vi "Read Serial Interface.vi"(8 "error in":errorcluster, 11 "VISA Interface in":refnum<class "VISA Interface.lvclass">) -> (0 "error out":errorcluster, 2 "Serial Interface":T1={"Baud Rate"=9600, "Data Bits "=8, "Parity"=enum."None", "Stop Bits"=0} {"Stop Bits" items=["1.0", "1.5", "2.0"]; "Baud Rate" items=["1200"=1200, "2400"=2400, "4800"=4800, "9600"=9600, "19200"=19200, "38400"=38400, "57600"=57600, "115200"=115200]}, 3 "VISA Interface out":refnum<class "VISA Interface.lvclass">)   [LabVIEW 2020, in "Plugin Instrument Driver.lvlib" / "VISA Interface.lvclass"]
doc: "Reads Serial Interface"
uses:
  VISA Interface.lvclass
  builds/Libraries/Shared GUI Library.lvlibp/Shared GUI Library/Instrument Settings/Interface/Serial Interafce.ctl
  VISA Interface.lvclass/VISA Interface.ctl
  builds/Libraries/Shared GUI Library.lvlibp
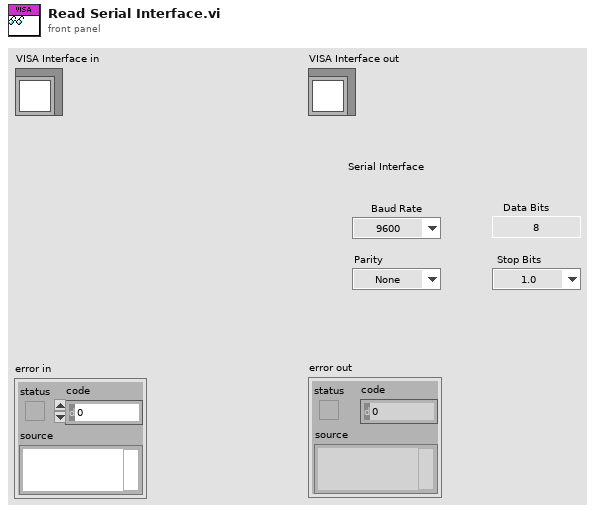
[diagram p1: front panel]
types:
  T1 = typedef "Shared GUI Library.lvlibp/Serial Interafce.ctl" = cluster{"Baud Rate":u32, "Data Bits ":u16, "Parity":enum16{"None", "Odd", "Even"}, "Stop Bits":u16}
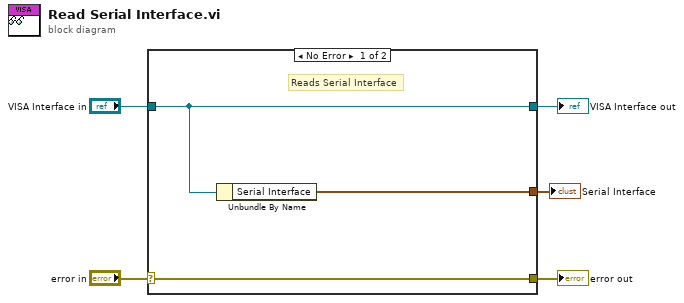
[diagram p0: block diagram]
diagram:
  n1 = case shown="No Error" "error in" {
    selector: "error in" -> [w8 w9]
    tunnel: [w8 w9] -> w4
    tunnel: [w7 w10] -> w2
    tunnel: "VISA Interface in" -> [w7 w10]
    tunnel: [w6 _] -> w1
    frame No Error {
      # "Reads Serial Interface"
      n2 = Unbundle By Name(w7) -> ("Serial Interface"=w6:T1)
    }
    frame Error {
    }
  }
  "error out" <- w4
  "VISA Interface out" <- w2
  "Serial Interface" <- w1
